vi "FTW-Test-JSON-Native.vi"() -> ()   [LabVIEW 2013]
uses:
  source/JSON/FTW-JSON-Core-LibraryFilepath.vi
  source/Reflection/FTW-Reflection-Type.vi
  source/JSON/FTW-JSON-Core-GetFlattenedValue.vi
  source/JSON/FTW-JSON-Core-LibraryError.vi
  source/CodeGen/JSON Deserialize/FTW-JSON-Deserialize.xnode
  source/JSON/FTW-JSON-Native-GetFlattenedValue.vi
  source/JSON/FTW-JSON-Validate.vi
panel:
  out "error out":errorcluster
  out "element":T1 {"subobject"."EXT" format="%_32g"; "subobject"."DBL" format="%_32g"; "subobject"."SGL" format="%_32g"; "EXT" format="%_32g"; "DBL" format="%_32g"; "SGL" format="%_32g"}
  in  "Object":string="{\n  \"booleanfalse\": false,\n  \"booleantrue\": true,\n  \"U8\": 8,\n  \"U16\": 16,\n  \"U32\": 32,\n  \"U64\": 64,\n  \"I8\": -8,\n  \"I16\": -16,\n  \"I32\": -32,\n  \"I64\": -64,\n  \"SGL\": 1.23456789,\n  \"DBL\": 1.2345678901234567,\n  \"EXT\": 1.2345678901234567,\n  \"nullstring\": null,\n  \"stringempty\": \"\",\n  \"stringHW\": \"Hello World\",\n  \"EnumU8\": \"U8\",\n  \"EnumU16\": \"U16\",\n  \"EnumU32\": \"U32\",\n  \"subobject\": {\n    \"booleanfalse\": false,\n    \"booleantrue\": true,\n    \"U8\": 8,\n    \"U16\": 16,\n    \"U32\": 32,\n    \"U64\": 64,\n    \"I8\": -8,\n    \"I16\": -16,\n    \"I32\": -32,\n    \"I64\": -64,\n    \"SGL\": 1.23456789,\n    \"DBL\": 1.2345678901234567,\n    \"EXT\": 1.2345678901234567,\n    \"nullstring\": null,\n    \"stringempty\": \"\",\n    \"stringHW\": \"Hello World\",\n    \"EnumU8\": \"U8\",\n    \"EnumU16\": \"U16\",\n    \"EnumU32\": \"U32\"\n  },\n  \"unusedpair\": \"whatever\"\n}"
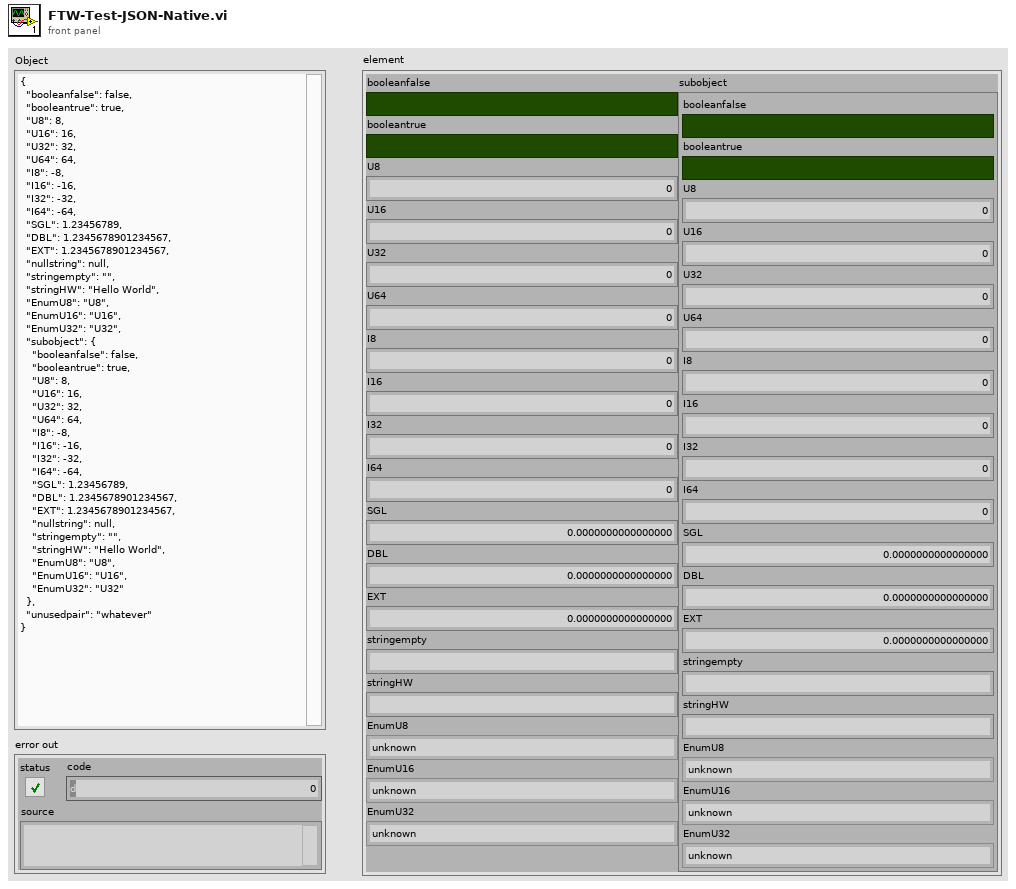
[diagram p1: front panel]
types:
  T1 = cluster{"booleanfalse":bool, "booleantrue":bool, "U8":u8, "U16":u16, "U32":u32, "U64":u64, "I8":i8, "I16":i16, "I32":i32, "I64":i64, "SGL":sgl, "DBL":dbl, "EXT":ext, "stringempty":string, "stringHW":string, "EnumU8":enum8{"unknown", "U8"}, "EnumU16":enum16{"unknown", "U16"}, "EnumU32":enum32{"unknown", "U32"}, "subobject":cluster{"booleanfalse":bool, "booleantrue":bool, "U8":u8, "U16":u16, "U32":u32, "U64":u64, "I8":i8, "I16":i16, "I32":i32, "I64":i64, "SGL":sgl, "DBL":dbl, "EXT":ext, "stringempty":string, "stringHW":string, "EnumU8":enum8{"unknown", "U8"}, "EnumU16":enum16{"unknown", "U16"}, "EnumU32":enum32{"unknown", "U32"}}}
  T2 = cluster{"booleanfalse":bool, "booleantrue":bool, "U8":u8, "U16":u16, "U32":u32, "U64":u64, "I8":i8, "I16":i16, "I32":i32, "I64":i64, "SGL":sgl, "DBL":dbl, "EXT":ext, "stringempty":string, "stringHW":string, "EnumU8":enum8{"unknown", "U8"}, "EnumU16":enum16{"unknown", "U16"}, "EnumU32":enum32{"unknown", "U32"}}
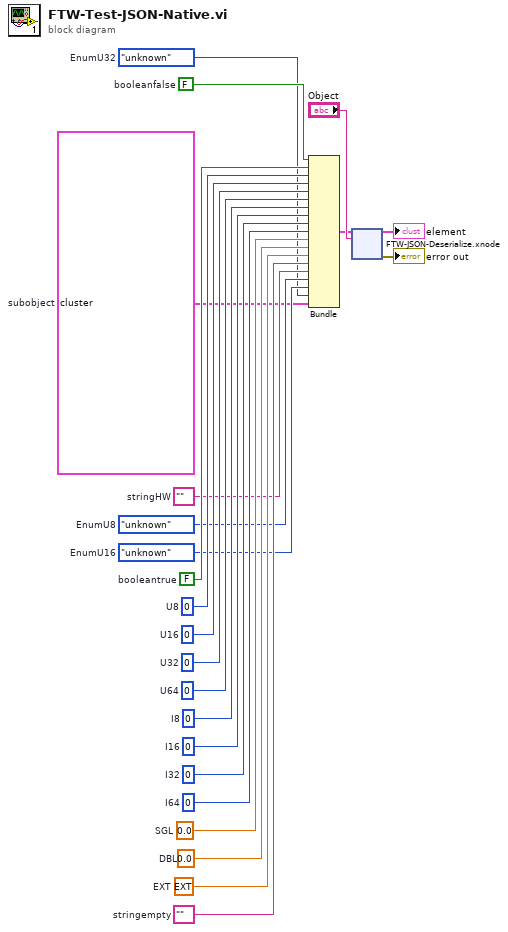
[diagram p0: block diagram]
diagram:
  w1 = T2 {"booleanfalse"=FALSE, "booleantrue"=FALSE, "U8"=0, "U16"=0, "U32"=0, "U64"=0, "I8"=0, "I16"=0, "I32"=0, "I64"=0, "SGL"=0.0, "DBL"=0.0, "EXT"=0.0, "stringempty"="", "stringHW"="", "EnumU8"=enum."unknown", "EnumU16"=enum."unknown", "EnumU32"=enum."unknown"}  # subobject
  w2 = enum32{"unknown", "U32"}."unknown"  # EnumU32
  w3 = enum16{"unknown", "U16"}."unknown"  # EnumU16
  w4 = enum8{"unknown", "U8"}."unknown"  # EnumU8
  w5 = ""  # stringHW
  w6 = ""  # stringempty
  w9 = FALSE  # booleantrue
  w10 = FALSE  # booleanfalse
  w11 = ext 0.0  # EXT
  w12 = 0.0  # DBL
  w13 = sgl 0.0  # SGL
  w14 = i64 0  # I64
  w15 = 0  # I32
  w16 = i16 0  # I16
  w17 = i8 0  # I8
  w18 = u64 0  # U64
  w19 = u32 0  # U32
  w20 = u16 0  # U16
  w21 = u8 0  # U8
  n1 = Bundle("booleanfalse"=w10, "booleantrue"=w9, "U8"=w21, "U16"=w20, "U32"=w19, "U64"=w18, "I8"=w17, "I16"=w16, "I32"=w15, "I64"=w14, "SGL"=w13, "DBL"=w12, "EXT"=w11, "stringempty"=w6, "stringHW"=w5, "EnumU8"=w4, "EnumU16"=w3, "EnumU32"=w2, "subobject"=w1) -> (w8:T1)  [unwired: 1 in]
  n2 = xnode "FTW-JSON-Deserialize.xnode"("Type and Defaults"=w8, "JSON String"="Object") -> ("Values"=→"element":T1, "error out"=→"error out":errorcluster)  [unwired: 1 in]
